vi "strChoiceArray.vi"() -> (0 "StrArray":string[](array[string])=["ValveCold", "ValveHot", "ValvePre", "WaterShot", "ValveBleach", "ValveDry", "ValveMist", "ValveSteam", "ValveChange", "ValveSoftener", "ValveFilter", "ValveActiveWash"], 1 "ColorArray":u32[](array[colorbox])=[16770560, 7995178, 2818039], 2 "大小":i32)   [LabVIEW 2011]
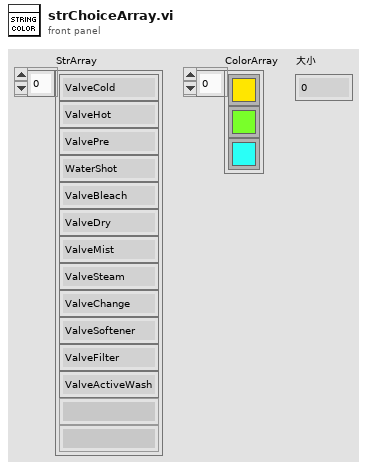
[diagram p1: front panel]
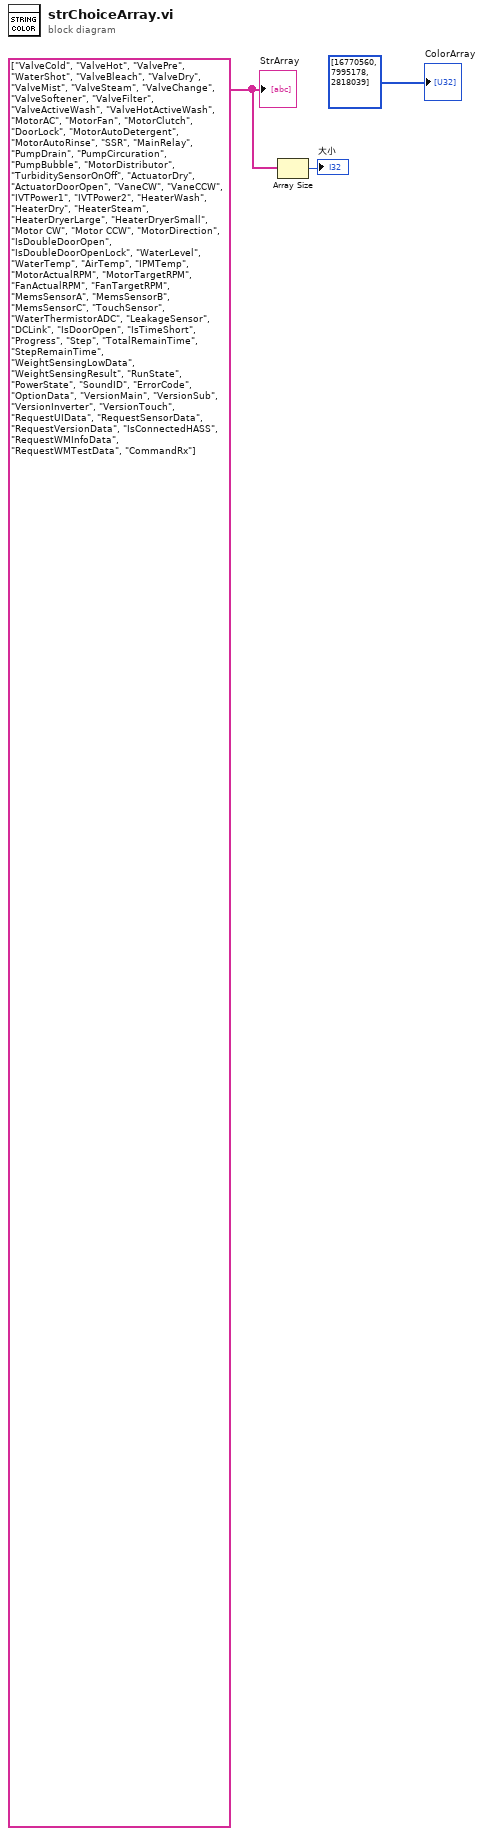
[diagram p0: block diagram]
diagram:
  w2 = string[] ["ValveCold", "ValveHot", "ValvePre", "WaterShot", "ValveBleach", "ValveDry", "ValveMist", "ValveSteam", "ValveChange", "ValveSoftener", "ValveFilter", "ValveActiveWash", "ValveHotActiveWash", "MotorAC", "MotorFan", "MotorClutch", "DoorLock", "MotorAutoDetergent", "MotorAutoRinse", "SSR", "MainRelay", "PumpDrain", "PumpCircuration", "PumpBubble", "MotorDistributor", "TurbiditySensorOnOff", "ActuatorDry", "ActuatorDoorOpen", "VaneCW", "VaneCCW", "IVTPower1", "IVTPower2", "HeaterWash", "HeaterDry", "HeaterSteam", "HeaterDryerLarge", "HeaterDryerSmall", "Motor CW", "Motor CCW", "MotorDirection", "IsDoubleDoorOpen", "IsDoubleDoorOpenLock", "WaterLevel", "WaterTemp", "AirTemp", "IPMTemp", "MotorActualRPM", "MotorTargetRPM", "FanActualRPM", "FanTargetRPM", "MemsSensorA", "MemsSensorB", "MemsSensorC", "TouchSensor", "WaterThermistorADC", "LeakageSensor", "DCLink", "IsDoorOpen", "IsTimeShort", "Progress", "Step", "TotalRemainTime", "StepRemainTime", "WeightSensingLowData", "WeightSensingResult", "RunState", "PowerState", "SoundID", "ErrorCode", "OptionData", "VersionMain", "VersionSub", "VersionInverter", "VersionTouch", "RequestUIData", "RequestSensorData", "RequestVersionData", "IsConnectedHASS", "RequestWMInfoData", "RequestWMTestData", "CommandRx"]
  n1 = Array Size(array=w2) -> (size(s)=→"大小":i32)
  "StrArray" <- w2
  "ColorArray" <- u32[] [16770560, 7995178, 2818039]
